vi "测量通道数转换scan list.vi"(1 "测量通道数":i32=2 min=1 max=100) -> (0 "Scan List":string)   [LabVIEW 2015]
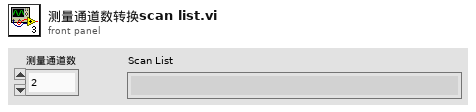
[diagram p1: front panel]
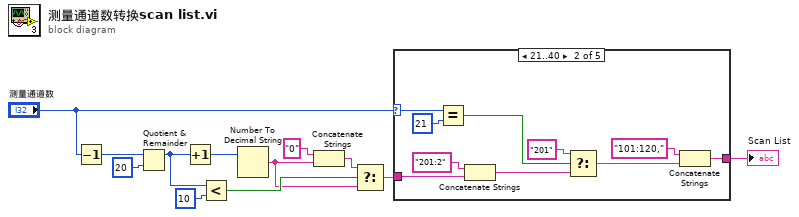
[diagram p0: block diagram]
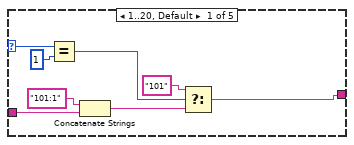
[diagram p2: hidden frame]
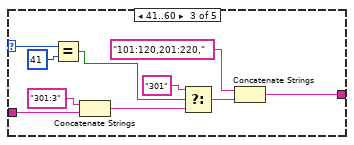
[diagram p3: hidden frame]
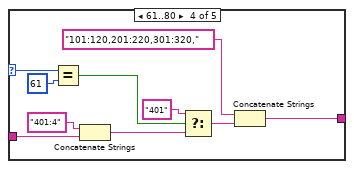
[diagram p4: hidden frame]
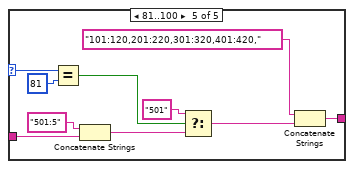
[diagram p5: hidden frame]
diagram:
  n1 = Decrement(x="测量通道数") -> (x-1=w2:i32)
  n2 = Quotient & Remainder(x=w2, y=20) -> (x-y*floor(x/y)=w7:i32)  [unwired: 1 out]
  n3 = Increment(x=w7) -> (x+1=w1:i32)
  n4 = Less?(x=w7, y=10) -> (x < y?=w9:bool)
  n5 = Number To Decimal String(number=w1) -> (decimal integer string=w5:string)  [unwired: 1 in]
  n6 = Concatenate Strings("0" ("Scan List"), w5) -> (w6:string)
  n7 = Select(t=w6, s=w9, f=w5) -> (s? t:f=w4:string)
  n8 = case shown="21..40" "测量通道数" {
    selector: "测量通道数" -> [w20 w30 w40 w50 w60]
    tunnel: w4 -> [w16 w26 w36 w46 w56]
    tunnel: [w13 w21 w31 w41 w51] -> w3
    frame 1..20, Default {
      n9 = Equal?(x=w20, y=1 ("slot")) -> (x = y?=w18:bool)
      n10 = Concatenate Strings("101:1" ("Scan List"), w16) -> (w14:string)
      n11 = Select(t="101" ("Scan List"), s=w18, f=w14) -> (s? t:f=w13:string)
    }
    frame 21..40 {
      n12 = Equal?(x=w30, y=21 ("slot")) -> (x = y?=w28:bool)
      n13 = Concatenate Strings("201:2" ("Scan List"), w26) -> (w24:string)
      n14 = Select(t="201" ("Scan List"), s=w28, f=w24) -> (s? t:f=w22:string)
      n15 = Concatenate Strings("101:120," ("Scan List"), w22) -> (w21:string)
    }
    frame 41..60 {
      n16 = Equal?(x=w40, y=41 ("slot")) -> (x = y?=w38:bool)
      n17 = Concatenate Strings("301:3" ("Scan List"), w36) -> (w34:string)
      n18 = Select(t="301" ("Scan List"), s=w38, f=w34) -> (s? t:f=w32:string)
      n19 = Concatenate Strings("101:120,201:220," ("Scan List"), w32) -> (w31:string)
    }
    frame 61..80 {
      n20 = Equal?(x=w50, y=61 ("slot")) -> (x = y?=w48:bool)
      n21 = Concatenate Strings("401:4" ("Scan List"), w46) -> (w44:string)
      n22 = Select(t="401" ("Scan List"), s=w48, f=w44) -> (s? t:f=w42:string)
      n23 = Concatenate Strings("101:120,201:220,301:320," ("Scan List"), w42) -> (w41:string)
    }
    frame 81..100 {
      n24 = Equal?(x=w60, y=81 ("slot")) -> (x = y?=w58:bool)
      n25 = Concatenate Strings("501:5" ("Scan List"), w56) -> (w54:string)
      n26 = Select(t="501" ("Scan List"), s=w58, f=w54) -> (s? t:f=w52:string)
      n27 = Concatenate Strings("101:120,201:220,301:320,401:420," ("Scan List"), w52) -> (w51:string)
    }
  }
  "Scan List" <- w3
